vi "SLIT_ROT_Write_Config.vi"(4 "error in (no error)":errorcluster, 7 "Config Refnum":T1) -> (0 "error out":errorcluster, 3 "refnum out":T1)   [LabVIEW 2015]
uses:
  <vilib>/Utility/config.llb/Config Data RefNum.ctl
  Systems/Slit/GSP_SLIT_Global.vi
  <vilib>/Utility/config.llb/Write Key (I32).vi
  <vilib>/Utility/config.llb/Write Key (Double).vi
  <vilib>/Utility/config.llb/NI_LVConfig.lvlib
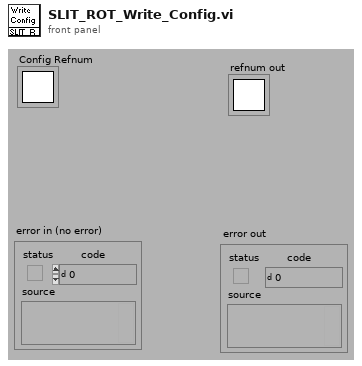
[diagram p1: front panel]
types:
  T1 = typedef "NI_LVConfig.lvlib/Config Data RefNum.ctl" = refnum<k1>
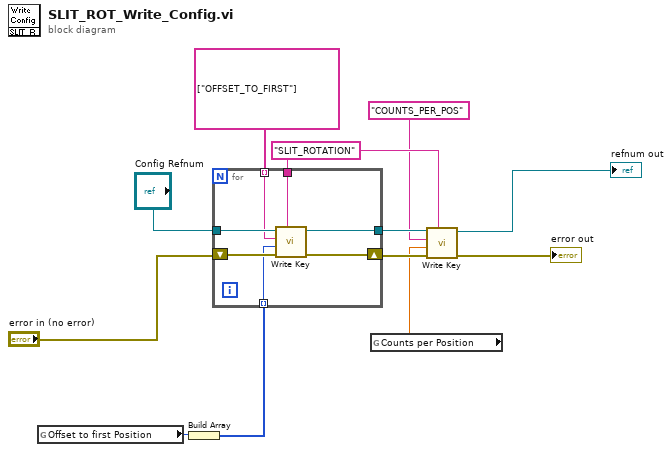
[diagram p0: block diagram]
diagram:
  w6 = "SLIT_ROTATION"
  n1 = global read "GSP_SLIT_Global.vi" "Offset to first Position"() -> (w1:i32)
  n2 = Build Array(w1) -> (w12:i32[])
  n3 = for {
    tunnel: "Config Refnum" -> [w18]
    shift-right: [w17] -> w7
    shift-left: "error in (no error)" -> [w19]
    tunnel: [w16] -> w8
    tunnel: w12 -> [w13] mode=indexing
    tunnel: string[] ["OFFSET_TO_FIRST"] -> [w15] mode=indexing
    tunnel: w6 -> [w14]
    n4 = call-poly <vilib>:"Write Key.vi"("section"=w14, "error in (no error)"=w19, "value"=w13, "key"=w15, "refnum"=w18) -> ("error out"=w17:errorcluster, "refnum out"=w16:T1)  [unwired: 4 in, 1 out]
  }
  n5 = global read "GSP_SLIT_Global.vi" "Counts per Position"() -> (w2:dbl)
  n6 = call-poly <vilib>:"Write Key.vi"("section"=w6, "error in (no error)"=w7, "value"=w2, "key"="COUNTS_PER_POS", "refnum"=w8) -> ("error out"=→"error out":errorcluster, "refnum out"=→"refnum out":T1)  [unwired: 4 in, 1 out]
